vi "(SubVI)I2C_16Bit-16Bit_Write_Sequential.vi"(5 "Log Ref":refnum<vi>, 7 "Clock":T1=enum."400kHz", 8 "error in (no error)":errorcluster caption="에러 입력(에러 없음)", 9 "Data to Write":u16[](array[numeric]), 10 "Start Address":u16, 11 "ID":u8) -> (0 "error out":errorcluster caption="에러 출력", 2 "Log":string)   [LabVIEW 2020]
uses:
  Controls/(Ctrl)I2C_Clock.ctl
  Controls/(Ctrl)I2C_RW.ctl
  Controls/(Ctrl)I2C_Data Size.ctl
  Serial/Controls/(Ctrl)Serial_Write Read Option.ctl
  Variables/(Var)System Variables.vi
  Serial/Instance VIs/(SubVI)Serial_Write-Read.vi
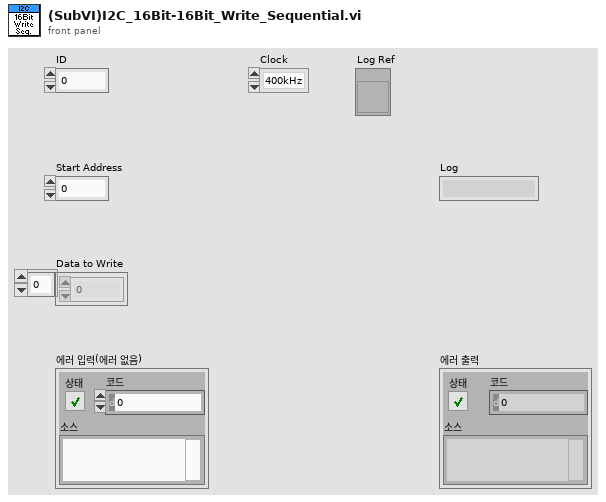
[diagram p1: front panel]
types:
  T1 = typedef "(Ctrl)I2C_Clock.ctl" = enum8{"1MHz", "2MHz", "3MHz", "400kHz"}
  T2 = typedef "(Ctrl)I2C_Data Size.ctl" = enum16{"8Bit_8Bit", "16Bit_16Bit", "16Bit_8Bit"}
  T3 = typedef "(Ctrl)I2C_RW.ctl" = enum16{"Read", "Write"}
  T4 = typedef "(Ctrl)Serial_Write Read Option.ctl" = cluster{"Echo Request":bool, "Header Verification":bool, "Checksum Verification":bool, "User Code Verifiaction":bool}
  T5 = typedef "IC I2C Clock Rate.ctl" = enum8{"50khz", "100khz", "400khz", "1Mhz", "1.2Mhz"}
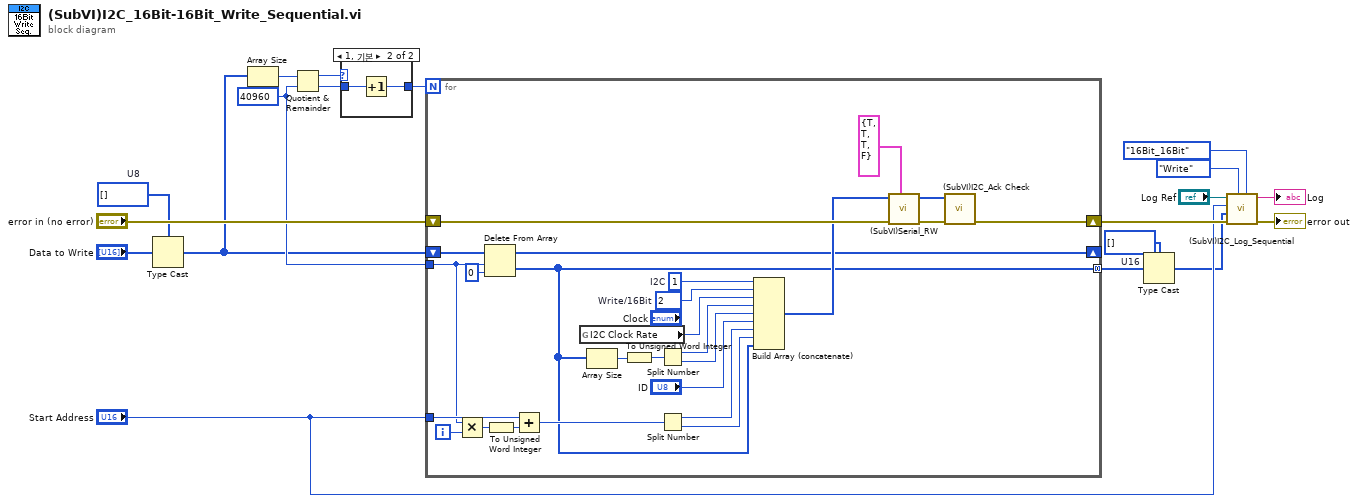
[diagram p0: block diagram]
diagram:
  w1 = u16[] []  # U16
  w3 = u8[] []  # U8
  w7 = 40960 ("y")
  n1 = Type Cast(type=w3, x="Data to Write") -> (*(type *) &x=w4:u8[])
  n2 = Array Size(array=w4) -> (size(s)=w11:i32)
  n3 = Quotient & Remainder(x=w11, y=w7) -> (x-y*floor(x/y)=w10:i32, floor(x/y)=w9:i32)
  n4 = case shown="1, 기본" w10 {
    tunnel: w9 -> [w20 w22]
    tunnel: [w20 w21] -> w8
    frame 0 {
    }
    frame 1, Default {
      n5 = Increment(x=w22) -> (x+1=w21:i32)
    }
  }
  n6 = for {
    N: w8 -> [_]
    tunnel: "Start Address" -> [w28]
    shift-right: [w40] -> w18
    shift-left: "error in (no error)" -> [w48]
    tunnel: w7 -> [w25]
    shift-right: [w31] -> _
    shift-left: w4 -> [w33]
    tunnel: [w24] -> w5 mode=concatenating
    i -> [w30]
    w45 = u8 2  # Write/16Bit
    w46 = u8 1  # I2C
    n7 = Multiply(x=w25, y=w30) -> (x*y=w29:i32)
    n8 = Delete From Array(array=w33, length=w25, index=0 ("인덱스")) -> (deleted portion=w24:u8[], array with subset deleted=w31:u8[])
    n9 = To Unsigned Word Integer(number=w29) -> (unsigned 16bit integer=w27:u16)
    n10 = Add(x=w28, y=w27) -> (x+y=w26:u16)
    n11 = global read "(Var)System Variables.vi" "I2C Clock Rate"() -> (w23:T5)
    n12 = Array Size(array=w24) -> (size(s)=w47:i32)
    n13 = To Unsigned Word Integer(number=w47) -> (unsigned 16bit integer=w41:u16)
    n14 = Split Number(x=w41) -> (hi(x)=w44:u8, lo(x)=w43:u8)
    n15 = Split Number(x=w26) -> (hi(x)=w38:u8, lo(x)=w39:u8)
    n16 = Build Array (concatenate)(w46, w45, w23, w44, w43, "ID", w38, w39, w24) -> (w34:u8[])
    n17 = call-poly "(SubVI)Serial_RW.vi"("Option"=T4 {"Echo Request"=TRUE, "Header Verification"=TRUE, "Checksum Verification"=TRUE, "User Code Verifiaction"=FALSE}, "error in (no error)"=w48, "Data to Write"=w34) -> ("error out"=w37:errorcluster, "Read Data"=w35:u8[])  [unwired: 6 in, 1 out]
    n18 = call "(SubVI)I2C_Ack Check.vi"("에러 입력(에러 없음)"=w37, "Read Data"=w35) -> ("에러 출력"=w40:errorcluster)  [unwired: 8 in, 1 out]
  }
  n19 = Type Cast(type=w1, x=w5) -> (*(type *) &x=w2:u16[])
  n20 = call "(SubVI)I2C_Log_Sequential.vi"("Data Size"=(Ctrl)I2C_Data_Size."16Bit_16Bit", "R/W"=(Ctrl)I2C_RW."Write", "error in (no error)"=w18, "Data Array"=w2, "Start Address"="Start Address", "Log Ref"="Log Ref") -> ("error out"=→"error out":errorcluster, "Log"=→"Log":string)  [unwired: 4 in]
